vi "KundtsTube.vi"() -> ()   [LabVIEW 2014]
uses:
  <vilib>/Utility/file.llb/Write To Spreadsheet File (DBL).vi
panel:
  out "XY Graph":cluster{"Y":dbl[], "Y":dbl[]}[](graph)=[{"Y"=[10.0, 15.0, 20.0, 25.0, 30.0, 35.0, 40.0, 45.0, 50.0, 55.0, 60.0, 65.0, 70.0, 75.0, 80.0, 85.0, 90.0, 95.0, 100.0, 105.0, 110.0, 115.0, 120.0, 125.0, 130.0, 135.0, 140.0, 145.0, 150.0, 155.0, 160.0, 165.0, 170.0, 175.0, 180.0, 185.0, 190.0, 195.0, 200.0, 205.0, 210.0, 215.0, 220.0, 225.0, 230.0, 235.0, 240.0, 245.0, 250.0, 255.0, 260.0, 265.0, 270.0, 275.0, 280.0, 285.0, 290.0, 295.0, 300.0, 305.0, 310.0, 315.0, 320.0, 325.0, 330.0, 335.0, 340.0, 345.0, 350.0, 355.0, 360.0, 365.0, 370.0, 375.0, 380.0, 385.0, 390.0, 395.0, 400.0, 405.0, 410.0, 415.0, 420.0, 425.0, 430.0, 435.0, 440.0, 445.0, 450.0, 455.0, 460.0, 465.0, 470.0, 475.0, 480.0, 485.0, 490.0, 495.0, 500.0, 505.0, 510.0, 515.0, 520.0, 525.0, 530.0, 535.0, 540.0, 545.0, 550.0, 555.0, 560.0, 565.0, 570.0, 575.0, 580.0, 585.0, 590.0, 595.0, 600.0, 605.0, 610.0, 615.0, 620.0, 625.0, 630.0, 635.0, 640.0, 645.0, 650.0, 655.0, 660.0, 665.0, 670.0, 675.0, 680.0, 685.0, 690.0, 695.0, 700.0, 705.0, 710.0, 715.0, 720.0, 725.0, 730.0, 735.0, 740.0, 745.0, 750.0, 755.0, 760.0, 765.0, 770.0, 775.0, 780.0, 785.0, 790.0, 795.0], "Y"=[0.006885423812333251, 0.003164409867754543, 0.006187733700200648, 0.007583113923322989, 0.005024916844106791, 0.007117987182790152, 0.007350550553120066, 0.008978494141873607, 0.027350999926165194, 0.032234830444175744, 0.014094888237437073, 0.033165083869815905, 0.015955395166032435, 0.02293229607581922, 0.02223460598998916, 0.022699732714003013, 0.024792802965771125, 0.026420746487802522, 0.03502559071498757, 0.03200226708744757, 0.039676857792275616, 0.040141984497203506, 0.0594447423023095, 0.0529329686830576, 0.058747052276457025, 0.06897983920722801, 0.2022386100083123, 0.10363177493180722, 0.1322370620132927, 0.17386589096366195, 0.2561932835450344, 0.43852281818524735, 0.8424847755772092, 0.6113171877816287, 0.35642802489465336, 0.24968151297047775, 0.1950291487935466, 0.1627028534370014, 0.1445629168242661, 0.12898117577662196, 0.1173530104404779, 0.10967842114311188, 0.11665532051011884, 0.09967819851609083, 0.09781769195472192, 0.09642231202832173, 0.09525949541947033, 0.09456180545262455, 0.11805070036968367, 0.10758535131053182, 0.10014332515515355, 0.10363177493180722, 0.10688766136403363, 0.11130636433905831, 0.11781813706007656, 0.1266555427350364, 0.13758601791894304, 0.15293519535807507, 0.16991231520687758, 0.1913081365051749, 0.22316930315478603, 0.2680540082590054, 0.3327065801708282, 0.43945307070674233, 0.6010844142335366, 0.7962047560860867, 0.7766694698679536, 0.5843398751440859, 0.4338715555462128, 0.3399160390050277, 0.28084498551356696, 0.2389836039489844, 0.21084345065070295, 0.18921506707846183, 0.17386589096366195, 0.17456358079923276, 0.15270263206771775, 0.19014532015829003, 0.13944652430499382, 0.13688832802205605, 0.1329347519178793, 0.1320044987115072, 0.13363244182131115, 0.13246962531494985, 0.13433013172358818, 0.13921396100718678, 0.14246984716480265, 0.14595829659146256, 0.15456313838697755, 0.16409823314404542, 0.17758690340664948, 0.19247095284883678, 0.21270395671230624, 0.2434023055345497, 0.30293849075507284, 0.3417765444902761, 0.41666188332471454, 0.5408505829006183, 0.719691546293932, 0.8517872914095912, 0.7513201089502469, 0.5671302092501487, 0.43247617674424754, 0.3457301186186972, 0.28619393952174327, 0.24596050116799006, 0.21572727904478303, 0.2103783241340109, 0.1794474096157815, 0.21944829111632386, 0.15805158771341668, 0.14828392952651429, 0.14060934079210347, 0.14107446738604865, 0.13619063812401394, 0.1352603849248277, 0.13014399229260498, 0.1299114289896649, 0.159912094009023, 0.1382837078146748, 0.13735345462010906, 0.14246984716480265, 0.149679309281379, 0.1606097838677537, 0.17061000504901302, 0.1864243078266038, 0.21061088739242148, 0.2399138569182497, 0.27898447975548885, 0.34712549771383927, 0.440383323226133, 0.641782943861708, 0.8522524171955062, 0.9069046932522183, 0.6557367245069972, 0.4629419461766887, 0.3478231872596479, 0.27828679009406715, 0.23154158012033038, 0.19875016104890517, 0.17479614407749888, 0.15805158771341668, 0.14572573329725091, 0.13456269502409055, 0.12712066934437954, 0.12316709314861372, 0.11525994064594113, 0.11223661759106714, 0.10991098445720272, 0.10758535131053182, 0.11316687084102653, 0.11293430752872884, 0.1108412377122854, 0.11409712408893634, 0.1175855737503413, 0.12456247298664476, 0.1285160491693309, 0.1399116509002228]}]
  out "Frequency":i32=795
  in  "Minimum Frequency":i32=10
  in  "Maximum Frequency":i32=10000
  in  "# of Points":i32=1999
  in  "Spacing":enum16{"Linear", "Logrithmic"}(ring)
  in  "Tab Control":enum32{"Sweep", "Single"}(tab)
  in  "Seconds to Wait":u32=1
  in  "Frequency":i32
  out "RMS":dbl=0.1399116509002228
  in  "# of Samples":dbl=10000.0
  in  "Sampling Rate":dbl=100000.0
  in  "Amplitude":i32=2
  in  "stop":bool
  out "Waveform Graph":dynamicdata(graph)=[{"t0"=timestamp(3498163829.3757586 s since 1904-01-01), "dt"=9.999999999999972e-06, "Y"=array[10000 elements], "attributes"=variant("NI_ChannelName"=variant(string "Voltage"), "NI_UnitDescription"=variant(string "Volts"))}]
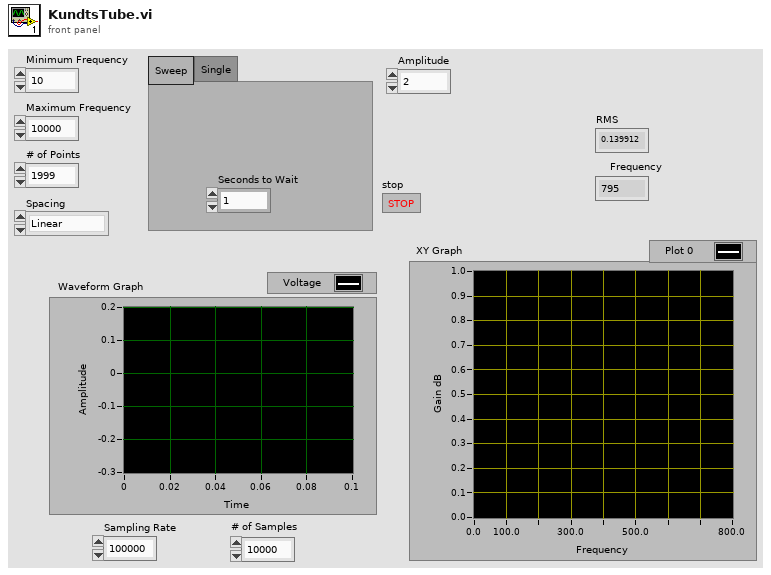
[diagram p1: front panel]
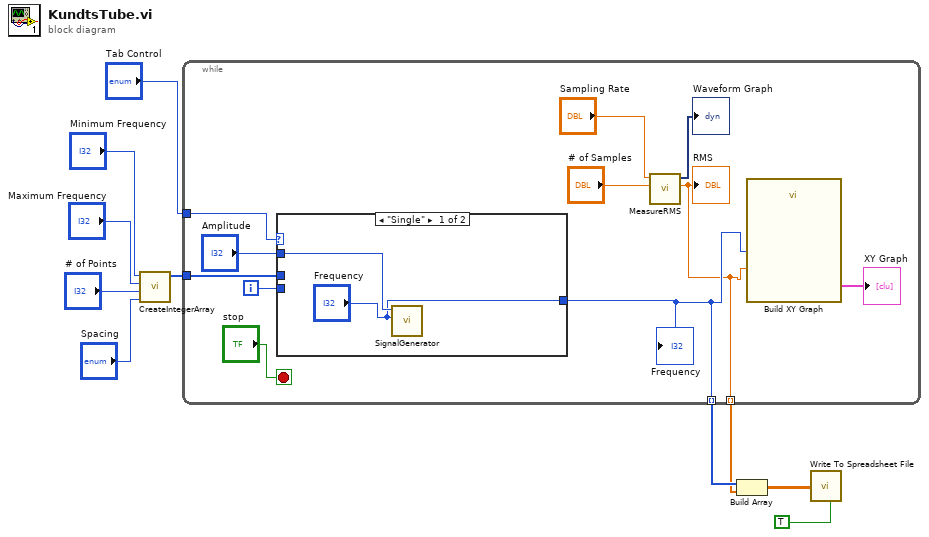
[diagram p0: block diagram]
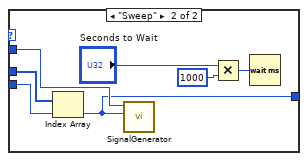
[diagram p2: hidden frame]
diagram:
  n1 = call "CreateIntegerArray.vi"("Spacing"="Spacing", "# of Points"="# of Points", "Maximum"="Maximum Frequency", "Minimum"="Minimum Frequency") -> ("Array"=w5:i32[])  [unwired: 7 in]
  n2 = while {
    tunnel: w5 -> [w15]
    tunnel: "Tab Control" -> [w18]
    tunnel: [w12] -> w3 mode=indexing
    tunnel: [w11] -> w2 mode=indexing
    i -> [w19]
    stop <- "stop" stop-if-true
    n3 = case shown="\"Single\"" w18 {
      tunnel: "Amplitude" -> [w23 w25]
      tunnel: w19 -> [_ w27]
      tunnel: w15 -> [_ w26]
      tunnel: ["Frequency" w24] -> w12
      frame "Single" {
        n4 = call "SignalGenerator.vi"("Frequency"="Frequency", "Amplitude"=w23) -> ()  [unwired: 9 in, 1 out]
      }
      frame "Sweep" {
        n5 = Index Array(array=w26, index=w27) -> (element=w24:i32)
        n6 = call "SignalGenerator.vi"("Frequency"=w24, "Amplitude"=w25) -> ()  [unwired: 9 in, 1 out]
        n7 = Multiply(x="Seconds to Wait", y=1000) -> (x*y=w30:u32)
        n8 = Wait (ms)(milliseconds to wait=w30) -> ()  [unwired: 1 out]
      }
    }
    "Frequency" <- w12
    n9 = call "MeasureRMS.vi"("Sampling Rate"="Sampling Rate", "# of Samples"="# of Samples") -> ("Waveform Graph"=→"Waveform Graph":dynamicdata, "RMS"=w11:dbl)  [unwired: 7 in]
    "RMS" <- w11
    n10 = call "Build XY Graph"("Y Input"=w11, "X Input"=w12) -> ("XY Graph"=→"XY Graph":cluster{"X":dbl[], "Y":dbl[]}[])  [unwired: 8 in, 1 out]
  }
  n11 = Build Array(w3, w2) -> (w1:dbl[][])
  n12 = call-poly <vilib>:"Write To Spreadsheet File.vi"("transpose? (no:F)"=TRUE, "2D data"=w1) -> ()  [unwired: 6 in, 1 out]
